vi "Render.vi"(8 "error in (no error)":errorcluster, 10 "String in":string, 11 "Bold in":refnum<class "Bold.lvclass">) -> (0 "error out":errorcluster, 2 "String out":string, 3 "Bold out":refnum<class "Bold.lvclass">)   [LabVIEW 2021, in "Markdown.lvlib" / "Bold.lvclass"]
uses:
  Bold.lvclass
  C:/GitHub/Markdown/src/Markdown/Markdown.lvclass
  BoldTag.vi
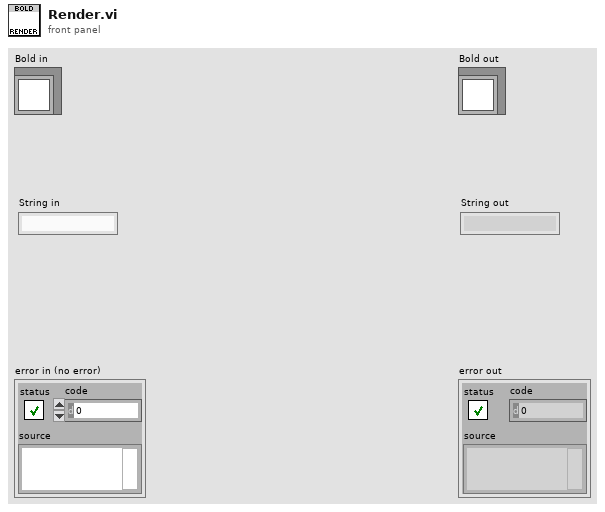
[diagram p1: front panel]
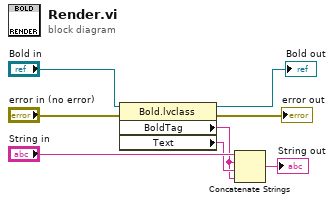
[diagram p0: block diagram]
diagram:
  n1 = property class="Bold.lvclass"(reference="Bold in", error in="error in (no error)") -> (reference out=→"Bold out":refnum<class "Bold.lvclass">, error out=→"error out":errorcluster, "BoldTag"=w6:string, "Text"=w7:string)
  n2 = Concatenate Strings("String in", w6, w7, w6) -> (→"String out":string)
